vi "Send Launch Event.vi"(8 "error in":errorcluster, 10 "Launch":bool, 11 "Engine in":refnum<class "Engine.lvclass">) -> (0 "error out":errorcluster, 3 "Engine out":refnum<class "Engine.lvclass">)   [LabVIEW 2023, in "Engine.lvlib" / "Engine.lvclass"]
doc: "Event used to trigger launch instructions from the Main UI to the Manual UI"
uses:
  Project/Engine.lvclass
  Project/Engine.lvclass/Engine.ctl
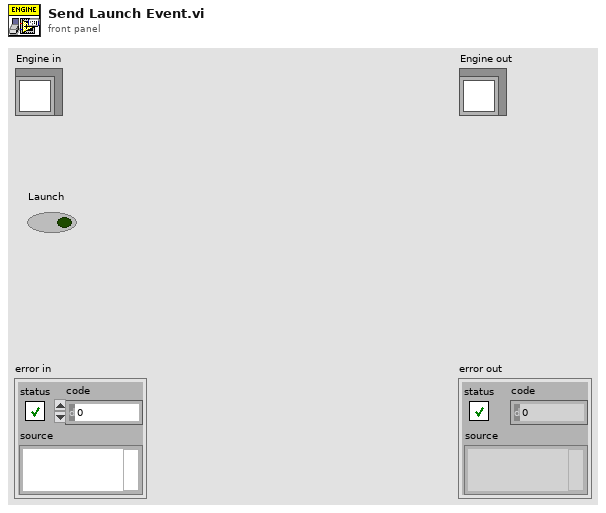
[diagram p1: front panel]
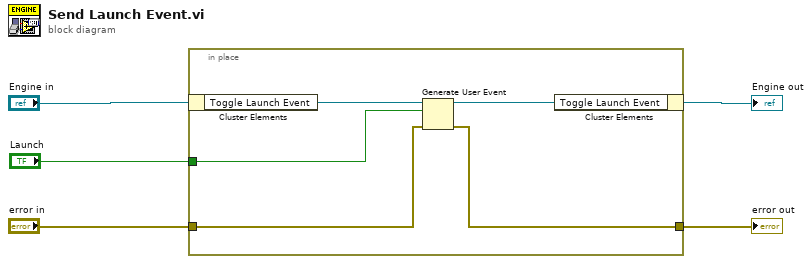
[diagram p0: block diagram]
diagram:
  n1 = in-place {
    in-place-border: "error in" -> [w8]
    in-place-border: [w7] -> w2
    in-place-border: "Launch" -> [w6]
    n2 = in-place-cluster #1("Engine in") -> ("Toggle Launch Event"=w10:refnum<user-event>)
    n3 = Generate User Event(user event=w10, event data cluster=w6, error in=w8) -> (user event out=w9:refnum<user-event>, error out=w7:errorcluster)  [unwired: 1 in]
    n4 = in-place-cluster #1("Toggle Launch Event"=w9) -> (→"Engine out":refnum<class "Engine.lvclass">)
  }
  "error out" <- w2
